vi "Remotely close panel.vi"(8 "error in (no error)":errorcluster, 10 "Clone name (blank = only one instance)":string, 11 "Fiber Auto Collimation panel in":refnum<class "Fiber Auto Collimation panel.lvclass">) -> (0 "error out":errorcluster, 3 "Fiber Auto Collimation panel out":refnum<class "Fiber Auto Collimation panel.lvclass">)   [LabVIEW 2018, in "Fiber Auto Collimation panel.lvclass"]
doc: "This VI sends an event to a panel instructing it to close, if it is open.\n\nThis VI will fail with no error if no instance of the panel is open, or if the clone name supplied doesn't match an open clone panel, or if no clone name is supplied and the panel class is clonable.\n\nThe incoming Panel type class will have its clone name set internally, and then that class will be sent as event data to the panel in question, so if any data needs to be sent to the panel as it is closing, write that data to the class wire before calling this VI.\n\nNote: The class data passed in will be identical to that which is passed out, the clone name input of this VI will not be on the wire."
uses:
  Fiber Auto Collimation panel.lvclass
  Fiber Auto Collimation panel.lvclass/Fiber Auto Collimation panel.ctl
  <vilib>/Utility/error.llb/Trim Whitespace.vi
  References/Fiber Auto Collimation References.lvclass
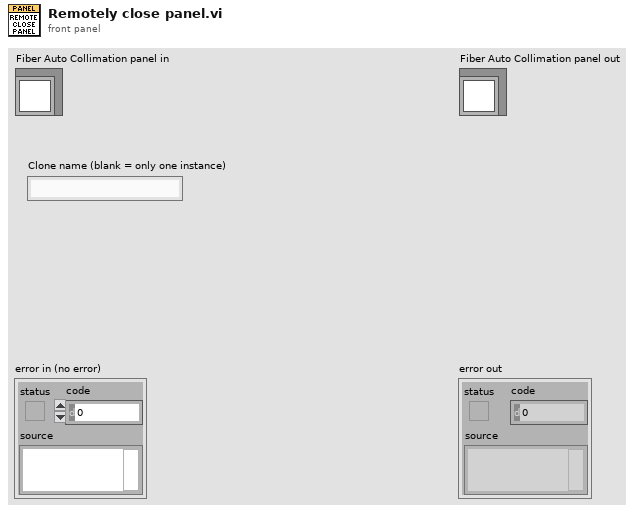
[diagram p1: front panel]
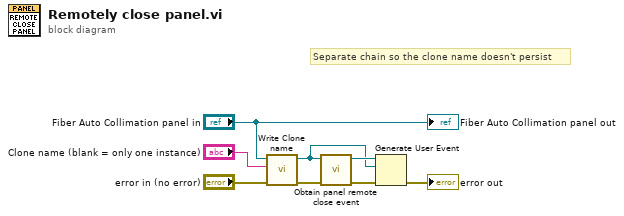
[diagram p0: block diagram]
diagram:
  # "Separate chain so the clone name doesn't persist"
  n1 = call "Write Clone name.vi"("error in (no error)"="error in (no error)", "Clone name"="Clone name (blank = only one instance)", "Fiber Auto Collimation panel in"="Fiber Auto Collimation panel in") -> ("error out"=w8:errorcluster, "Fiber Auto Collimation panel out"=w2:refnum<class "Fiber Auto Collimation panel.lvclass">)  [unwired: 7 in]
  n2 = call "Obtain panel remote close event.vi"("error in (no error)"=w8, "Fiber Auto Collimation panel"=w2) -> ("error out"=w5:errorcluster, "Panel remote close"=w4:refnum<user-event>)  [unwired: 8 in]
  n3 = Generate User Event(user event=w4, event data cluster=w2, error in=w5) -> (error out=→"error out":errorcluster)  [unwired: 1 in, 1 out]
  "Fiber Auto Collimation panel out" <- "Fiber Auto Collimation panel in"
